vi "Realsense Cam Disconnect.vi"(8 "error in (no error)":errorcluster, 11 "Realsense Cam in":refnum<class "Realsense Cam.lvclass">) -> (0 "error out":errorcluster, 3 "Realsense Cam out":refnum<class "Realsense Cam.lvclass">)   [LabVIEW 2018, in "Realsense Cam.lvclass"]
uses:
  Realsense Cam.lvclass
  Realsense Cam.lvclass/Realsense Cam.ctl
  Temp/realsense_labview_sdk/RealSense SDK2.11.0 for LabVIEW/libRealSense3.lvlib
panel:
  out "Close Error":string="No Error\rNo Error\rNo Error\rNo Error"
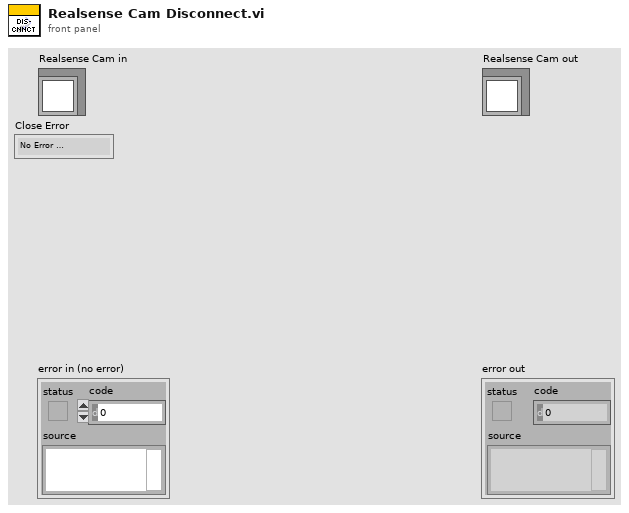
[diagram p1: front panel]
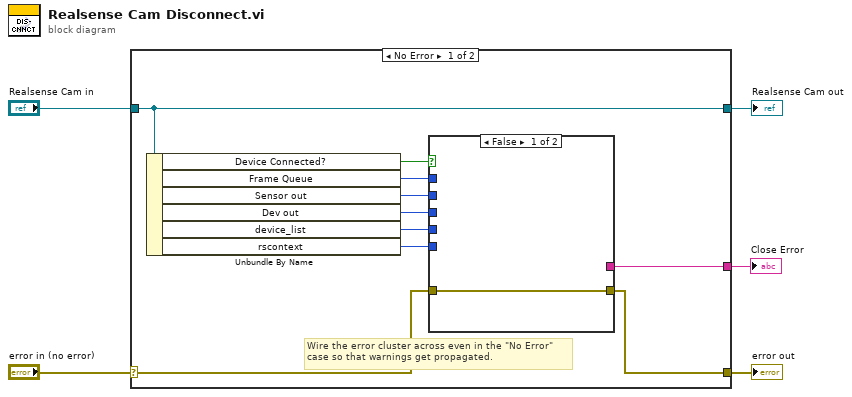
[diagram p0: block diagram]
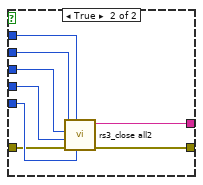
[diagram p2: hidden frame]
diagram:
  n1 = case shown="No Error" "error in (no error)" {
    selector: "error in (no error)" -> [w10 w26]
    tunnel: [w9 w26] -> w4
    tunnel: [w6 w25] -> w2
    tunnel: "Realsense Cam in" -> [w6 w25]
    tunnel: [w8 _] -> w1
    frame No Error {
      # "Wire the error cluster across even in the \"No Error\"\ncase so that warnings get propagated."
      n2 = Unbundle By Name(w6) -> ("Device Connected?"=w7:bool, "Frame Queue"=w15:u64, "Sensor out"=w14:u64, "Dev out"=w13:u64, "device_list"=w12:u64, "rscontext"=w11:u64)
      n3 = case shown="False" w7 {
        tunnel: w15 -> [_ w24]
        tunnel: w14 -> [_ w23]
        tunnel: w13 -> [_ w22]
        tunnel: w12 -> [_ w21]
        tunnel: w11 -> [_ w20]
        tunnel: w10 -> [w16 w19]
        tunnel: [w16 w18] -> w9
        tunnel: [_ w17] -> w8
        frame False {
        }
        frame True {
          n4 = call "rs3_close all2.vi"("rscontext"=w20, "queue in"=w24, "error in (no error)"=w19, "device_list"=w21, "Dev in"=w22, "Sensor in"=w23) -> ("error out (no error)"=w18:errorcluster, "Close Error"=w17:string)  [unwired: 4 in]
        }
      }
    }
    frame Error {
    }
  }
  "error out" <- w4
  "Realsense Cam out" <- w2
  "Close Error" <- w1
